vi "4bar Contol Loop.vi"() -> ()   [LabVIEW 2018]
uses:
  <vilib>/Rock Robotics/WPI/ThirdParty/Phoenix-LabVIEW/Motor Controller/Controls/CTRE_Phoenix_MotorControl_NeutralMode.ctl
  Infrastructure/RobotMap.vi
  Infrastructure/Constants.vi
  <vilib>/Rock Robotics/WPI/Switch/WPI_SwitchOpenLimit.vi
  Robot Global Data.vi
  <vilib>/Rock Robotics/WPI/ThirdParty/Phoenix-LabVIEW/Motor Controller/Get/CTRE_Phoenix_MotorController_GetSelectedSensorData.vi
panel:
  out "4bar Velocity":i32(graph)
  out "4bar Position":i32(graph)
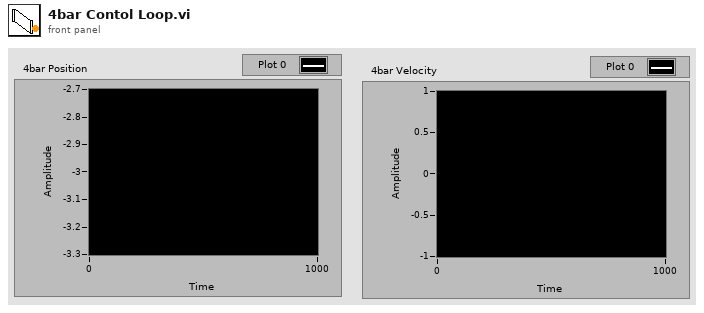
[diagram p1: front panel]
types:
  T1 = typedef "CTRE_Phoenix_MotorControl_NeutralMode.ctl" = enum8{"EEPROMSetting", "Override to Coast", "Override to Brake"}
  T2 = typedef "WPI_MotorControlDeviceRef.ctl" = cluster{"DeviceStatus":errorcluster, "Type":T3, "PWM":cluster{"PWM Channel":T4, "DeadBand":T5}, "CAN":cluster{"Device Number":u8, "SetOutput VI Ref":variant, "GetOutput VI Ref":variant, "Enable VI Ref":variant, "Disable VI Ref":variant, "Data":variant}, "Invert":bool, "DIO PWM":cluster{"PWM \"Enable\" Channel":T4, "DIOChannel":T6, "PWM Rate":dbl}}
  T3 = typedef "WPI_MotorControlType.ctl" = enum16{"PWM", "CAN", "DIO PWM"}
  T4 = typedef "FPGA_DIOPWMChannel.ctl" = enum8{"PWM 0", "PWM 1", "PWM 2", "PWM 3", "PWM 4", "PWM 5", "PWM 6", "PWM 7", "PWM 8", "PWM 9", "PWM MXP 0", "PWM MXP 1", "PWM MXP 2", "PWM MXP 3", "PWM MXP 4", "PWM MXP 5", "PWM MXP 6", "PWM MXP 7", "PWM MXP 8", "PWM MXP 9", "Invalid"}
  T5 = typedef "WPI_PWMDeadband.ctl" = cluster{"Name":string, "maxPositivePwm":i32, "minPositivePwm":i32, "centerPwm":i32, "maxNegativePwm":i32, "minNegativePwm":i32, "angularRange":u16}
  T6 = typedef "FPGA_DIOChannel.ctl" = enum8{"DIO 0", "DIO 1", "DIO 2", "DIO 3", "DIO 4", "DIO 5", "DIO 6", "DIO 7", "DIO 8", "DIO 9", "DIO MXP 0", "DIO MXP 1", "DIO MXP 2", "DIO MXP 3", "DIO MXP 4", "DIO MXP 5", "DIO MXP 6", "DIO MXP 7", "DIO MXP 8", "DIO MXP 9", "DIO MXP 10", "DIO MXP 11", "DIO MXP 12", "DIO MXP 13", "DIO MXP 14", "DIO MXP 15", "SPI Port CS1", "SPI Port CS2", "SPI Port CS3", "SPI Port MISO", "SPI Port MOSI", "Invalid"}
  T7 = typedef "WPI_SwitchDevRef.ctl" = cluster{"DevStatus":errorcluster, "DIO Channel":T6, "CntIndex":T8, "Normally Closed":bool}
  T8 = typedef "FPGA_CounterCtrSystemIndex.ctl" = enum8{"Ctr 0", "Ctr 1", "Ctr 2", "Ctr 3", "Ctr 4", "Ctr 5", "Ctr 6", "Ctr 7", "Invalid"}
  T9 = cluster{"P":dbl, "I":dbl, "D":dbl, "F":dbl, "I Zone":dbl}
  T10 = cluster{"Cruise Velocity":i32, "Acceleration":i32}
  T11 = typedef "CTRE_Phoenix_MotorControl_ControlMode.ctl" = u16
  T12 = cluster{"Control Mode":T11, "Operator Right Joystick Y out":dbl}
  T13 = cluster{"Position (Raw Sensor Units)":i32, "Velocity (Raw Sensor Units per 100 ms)":i32}
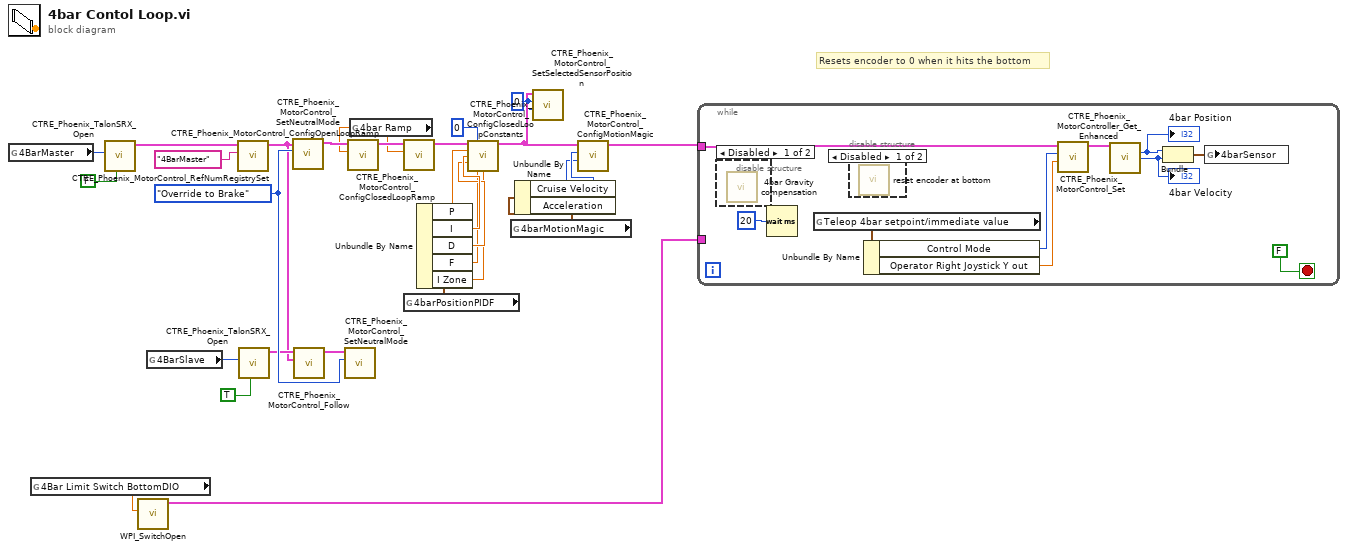
[diagram p0: block diagram]
diagram:
  w1 = 0 ("New Sensor Position")
  w29 = CTRE_Phoenix_MotorControl_NeutralMode."Override to Brake" ("Motor Control Neutral Mode")
  # "Resets encoder to 0 when it hits the bottom"
  n1 = global read "RobotMap.vi" "4BarMaster"() -> (w21:u8)
  n2 = global read "RobotMap.vi" "4Bar Limit Switch BottomDIO"() -> (w22:dbl)
  n3 = call <vilib>:"CTRE_Phoenix_TalonSRX_Open.vi"("Invert"=FALSE, "Device Number"=w21) -> ("CAN Talon SRX Ref"=w26:T2)  [unwired: 8 in, 1 out]
  n4 = call-poly <vilib>:"WPI_SwitchOpen.vi"("DIO Channel"=w22) -> ("SwitchDevRef"=w23:T7)  [unwired: 9 in, 1 out]
  n5 = global read "RobotMap.vi" "4BarSlave"() -> (w20:u8)
  n6 = call <vilib>:"CTRE_Phoenix_MotorControl_RefNumRegistrySet.vi"("refnum name"="4BarMaster", "PhoenixMotorControlDevRef"=w26) -> ("PhoenixMotorControlDevRef"=w9:T2)  [unwired: 8 in, 1 out]
  n7 = call <vilib>:"CTRE_Phoenix_TalonSRX_Open.vi"("Invert"=TRUE, "Device Number"=w20) -> ("CAN Talon SRX Ref"=w24:T2)  [unwired: 8 in, 1 out]
  n8 = call <vilib>:"CTRE_Phoenix_MotorControl_SetNeutralMode.vi"("Motor Control Neutral Mode"=w29, "PhoenixMotorControlDevRef"=w9) -> ("PhoenixMotorControlDevRef"=w25:T2)  [unwired: 8 in, 1 out]
  n9 = call <vilib>:"CTRE_Phoenix_MotorControl_Follow.vi"("Master Controller to Follow"=w9, "PhoenixMotorControlDevRef"=w24) -> ("PhoenixMotorControlDevRef"=w28:T2)  [unwired: 8 in, 1 out]
  n10 = call <vilib>:"CTRE_Phoenix_MotorControl_SetNeutralMode.vi"("Motor Control Neutral Mode"=w29, "PhoenixMotorControlDevRef"=w28) -> ()  [unwired: 8 in, 2 out]
  n11 = global read "Constants.vi" "4bar Ramp"() -> (w18:dbl)
  n12 = call <vilib>:"CTRE_Phoenix_MotorControl_ConfigOpenLoopRamp.vi"("secondsFromNeutralToFull"=w18, "PhoenixMotorControlDevRef"=w25) -> ("PhoenixMotorControlDevRef"=w19:T2)  [unwired: 8 in, 1 out]
  n13 = call <vilib>:"CTRE_Phoenix_MotorControl_ConfigClosedLoopRamp.vi"("secondsFromNeutralToFull"=w18, "PhoenixMotorControlDevRef"=w19) -> ("PhoenixMotorControlDevRef"=w11:T2)  [unwired: 8 in, 1 out]
  n14 = global read "Constants.vi" "4barPositionPIDF"() -> (w17:T9)
  n15 = Unbundle By Name(w17) -> ("P"=w16:dbl, "I"=w15:dbl, "D"=w14:dbl, "F"=w13:dbl, "I Zone"=w12:dbl)
  n16 = call <vilib>:"CTRE_Phoenix_MotorControl_ConfigClosedLoopConstants.vi"("PhoenixMotorControlDevRef"=w11, "slotIdx"=0, "P"=w16, "I"=w15, "D"=w14, "F"=w13, "I Zone"=w12) -> ("PhoenixMotorControlDevRef"=w2:T2)  [unwired: 7 in, 1 out]
  n17 = global read "Constants.vi" "4barMotionMagic"() -> (w5:T10)
  n18 = Unbundle By Name(w5) -> ("Cruise Velocity"=w4:i32, "Acceleration"=w3:i32)
  n19 = call <vilib>:"CTRE_Phoenix_MotorControl_SetSelectedSensorPosition.vi"("pidLoopIdx"=w1, "New Sensor Position"=w1, "PhoenixMotorControlDevRef"=w2) -> ()  [unwired: 7 in, 2 out]
  n20 = call <vilib>:"CTRE_Phoenix_MotorControl_ConfigMotionMagic.vi"("Acceleration"=w3, "Cruise Velocity"=w4, "PhoenixMotorControlDevRef"=w2) -> ("PhoenixMotorControlDevRef"=w6:T2)  [unwired: 7 in, 1 out]
  n21 = while {
    tunnel: w6 -> [w30]
    tunnel: w23 -> [_]
    stop <- FALSE stop-if-true
    n22 = disable-structure shown="Disabled" {
      frame Disabled {
        n23 = call "4bar Gravity compensation.vi"() -> ()  [unwired: 11 in, 1 out]
      }
      frame Enabled {
      }
    }
    n24 = Wait (ms)(milliseconds to wait=u32 20) -> ()  [unwired: 1 out]
    n25 = global read "Robot Global Data.vi" "Teleop 4bar setpoint/immediate value"() -> (w33:T12)
    n26 = disable-structure shown="Disabled" {
      frame Disabled {
        n27 = call "reset encoder at bottom.vi"() -> ()  [unwired: 11 in, 1 out]
      }
      frame Enabled {
      }
    }
    n28 = Unbundle By Name(w33) -> ("Control Mode"=w37:T11, "Operator Right Joystick Y out"=w34:dbl)
    n29 = call <vilib>:"CTRE_Phoenix_MotorControl_Set.vi"("Output"=w34, "Control Mode"=w37, "PhoenixMotorControlDevRef"=w30) -> ("PhoenixMotorControlDevRef"=w36:T2)  [unwired: 7 in, 1 out]
    n30 = call-poly <vilib>:"CTRE_Phoenix_MotorController_Get_Enhanced.vi"("PhoenixMotorControlDevRef"=w36) -> ("Position (Raw Sensor Units)"=w32:i32, "Velocity (Raw Sensor Units per 100 ms)"=w31:i32)  [unwired: 11 in, 2 out]
    "4bar Position" <- w32
    "4bar Velocity" <- w31
    n31 = Bundle("Position (Raw Sensor Units)"=w32, "Velocity (Raw Sensor Units per 100 ms)"=w31) -> (w35:T13)  [unwired: 1 in]
    n32 = global write "Robot Global Data.vi" "4barSensor"(w35) -> ()
  }
